vi "Re-Set Start Time.vi"(8 "error in (no error)":errorcluster, 10 "New Start Time":timestamp format="%<%x %.3X>T", 11 "Time Entries in":refnum<class "Time Entries.lvclass">) -> (0 "error out":errorcluster, 2 "Initial Display":string[](array[string]), 3 "Time Entries out":refnum<class "Time Entries.lvclass">)   [LabVIEW 2020, in "Time Entries.lvclass"]
doc: "Sets the new time as the start time for the Time Entry. Automatically recalculates the time entry for display.\n\n04/2025 Erich Schlieper"
uses:
  Time Entries.lvclass
  Time Entries.lvclass/Time Entries.ctl
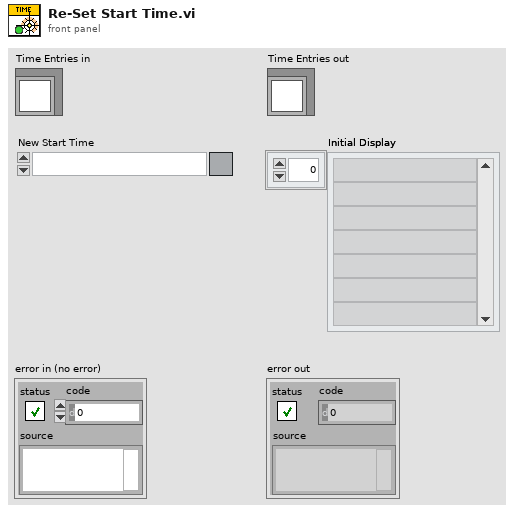
[diagram p1: front panel]
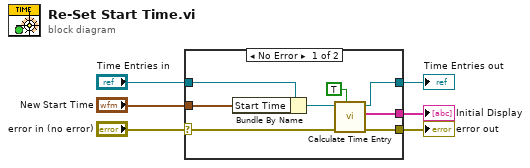
[diagram p0: block diagram]
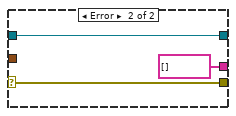
[diagram p2: hidden frame]
diagram:
  n1 = case shown="No Error" "error in (no error)" {
    selector: "error in (no error)" -> [w10 w17]
    tunnel: [w9 w17] -> w5
    tunnel: [w8 w16] -> w3
    tunnel: "Time Entries in" -> [w14 w16]
    tunnel: "New Start Time" -> [w13 _]
    tunnel: [w11 string[] [] ("Initial Display")] -> w1
    frame No Error {
      n2 = Bundle By Name(cluster=w14, "Start Time"=w13) -> (w7:refnum<class "Time Entries.lvclass">)
      n3 = call-dynamic "Calculate Time Entry.vi"("Recalculate Override (F)"=TRUE, "error in (no error)"=w10, "Time Entries in"=w7) -> ("error out"=w9:errorcluster, "Initial Display"=w11:string[], "Time Entries out"=w8:refnum<class "Time Entries.lvclass">)  [unwired: 6 in]
    }
    frame Error {
    }
  }
  "error out" <- w5
  "Time Entries out" <- w3
  "Initial Display" <- w1
